vi "tearDown.vi"(8 "error in (no error)":errorcluster, 11 "reference in":refnum<class "BC Major Frame.lvclass">) -> (0 "error out":errorcluster, 3 "reference out":refnum<class "BC Major Frame.lvclass">)   [LabVIEW 2016, in "BC Major Frame.lvclass"]
doc: "tearDown runs after the test method has completed. Use this method to clean up any operations or references that were opened by setUp or the test method. Unit tests should be independent of other unit tests so this VI should ensure that the next test can run in a 'clean' test environment."
uses:
  BC Major Frame.lvclass
  BC Major Frame.lvclass/BC Major Frame.ctl
  <vilib>/Utility/error.llb/Clear Errors.vi
  Dependencies/Registry/Registry.lvclass
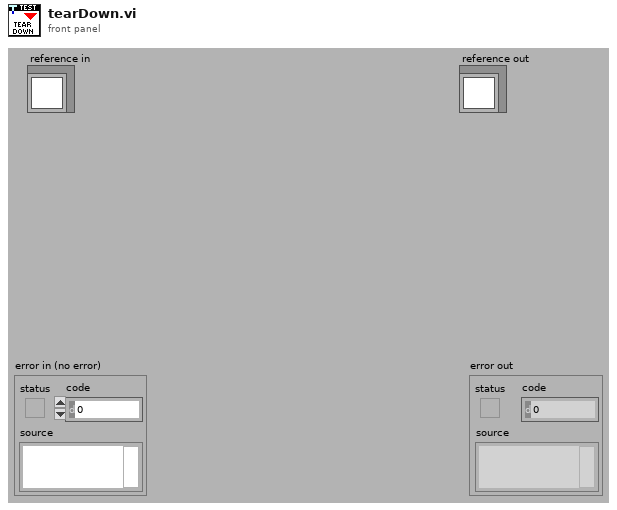
[diagram p1: front panel]
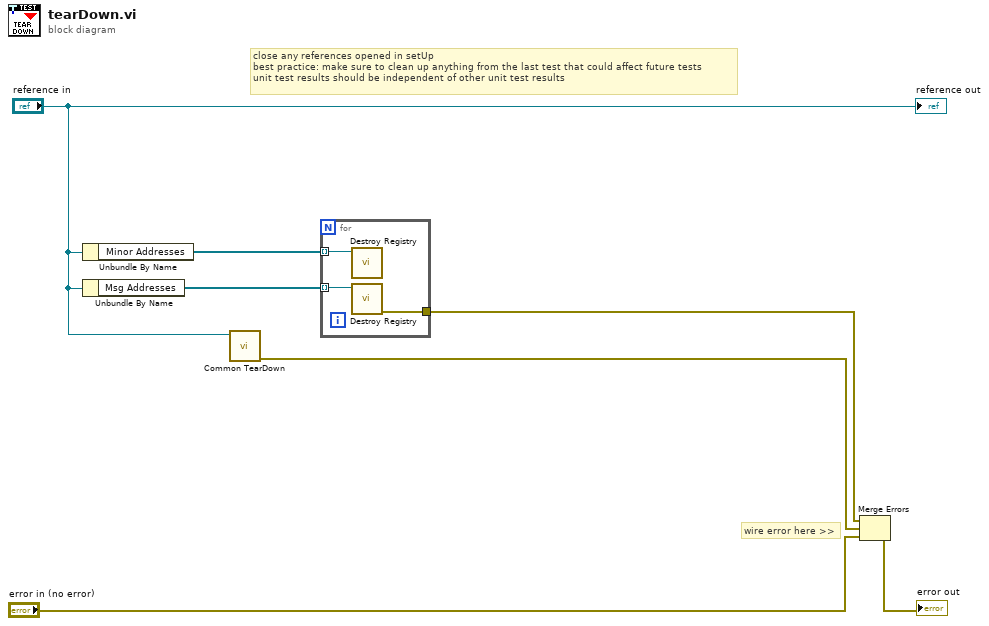
[diagram p0: block diagram]
diagram:
  # "wire error here >>"
  # "close any references opened in setUp\nbest practice: make sure to clean up anything from the last test that could affect future tests\nunit test results should be independent of other unit test results"
  n1 = Unbundle By Name("reference in") -> ("Minor Addresses"=w1:refnum<class "Registry.lvclass">[])
  n2 = Unbundle By Name("reference in") -> ("Msg Addresses"=w3:refnum<class "Registry.lvclass">[])
  n3 = call-dynamic "Common TearDown.vi"("1553 Test in"="reference in") -> ("error out"=w5:errorcluster)  [unwired: 9 in, 1 out]
  n4 = for {
    tunnel: [w10] -> w4
    tunnel: w3 -> [w9] mode=indexing
    tunnel: w1 -> [w8] mode=indexing
    n5 = call "Destroy Registry.vi"("Registry in"=w8) -> ()  [unwired: 7 in, 4 out]
    n6 = call "Destroy Registry.vi"("Registry in"=w9) -> ("error out"=w10:errorcluster)  [unwired: 7 in, 3 out]
  }
  n7 = Merge Errors(w4, w5, "error in (no error)") -> (→"error out":errorcluster)
  "reference out" <- "reference in"
